vi "FindSlide.vi"(0 "LUT":T1(array[cluster]), 1 "Mouse Position":cluster{"X":i32, "Y":i32}) -> (2 "slide":i32, 4 "position":T2)   [LabVIEW 2014]
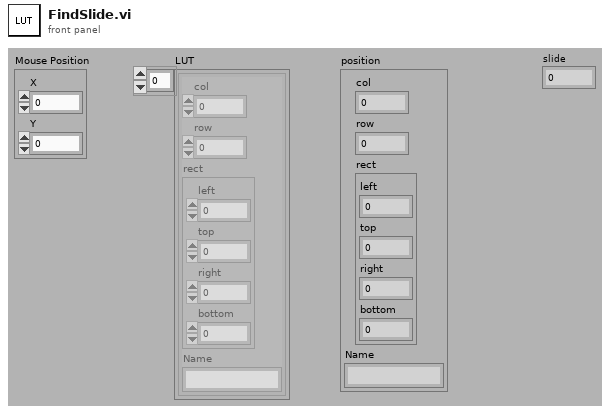
[diagram p1: front panel]
types:
  T1 = cluster{"col":i32, "row":i32, "rect":cluster{"left":i16, "top":i16, "right":i16, "bottom":i16}, "Name":string}[]
  T2 = cluster{"col":i32, "row":i32, "rect":cluster{"left":i16, "top":i16, "right":i16, "bottom":i16}, "Name":string}
  T3 = cluster{"left":i16, "top":i16, "right":i16, "bottom":i16}
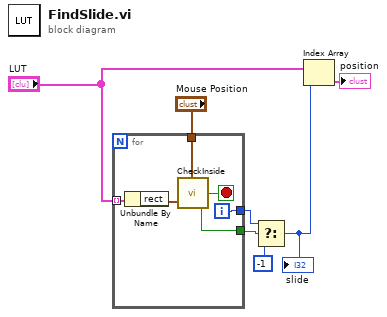
[diagram p0: block diagram]
diagram:
  n1 = for {
    tunnel: "LUT" -> [w12] mode=indexing
    tunnel: "Mouse Position" -> [w11]
    tunnel: [w10] -> w3
    tunnel: [w9] -> w4
    i -> [w10]
    stop <- w9 stop-if-true
    n2 = Unbundle By Name(w12) -> ("rect"=w8:T3)
    n3 = call "CheckInside.vi"("rect"=w8, "Coords"=w11) -> ("Inside?"=w9:bool)
  }
  n4 = Select(t=w3, s=w4, f=-1) -> (s? t:f=w7:i32)
  "slide" <- w7
  n5 = Index Array(array="LUT", index=w7) -> (element=→"position":T2)
